vi "UpdateCurveSetup.vi"(8 "ErrorIn(No Error)":errorcluster caption="entrée d'erreur (pas d'erreur)", 10 "CurveSetupsIn":T1[](array[typedef]), 11 "Interface.lvclass":refnum<class "Interface.lvclass">) -> (0 "sortie d'erreur":errorcluster, 3 "Interface.lvclass Out":refnum<class "Interface.lvclass">)   [LabVIEW 2019, in "Interface.lvclass"]
uses:
  Interface.lvclass
  CurveSetup.ctl
  Interface.lvclass/Interface.ctl
panel:
  # "Chemin de sauvegarde"
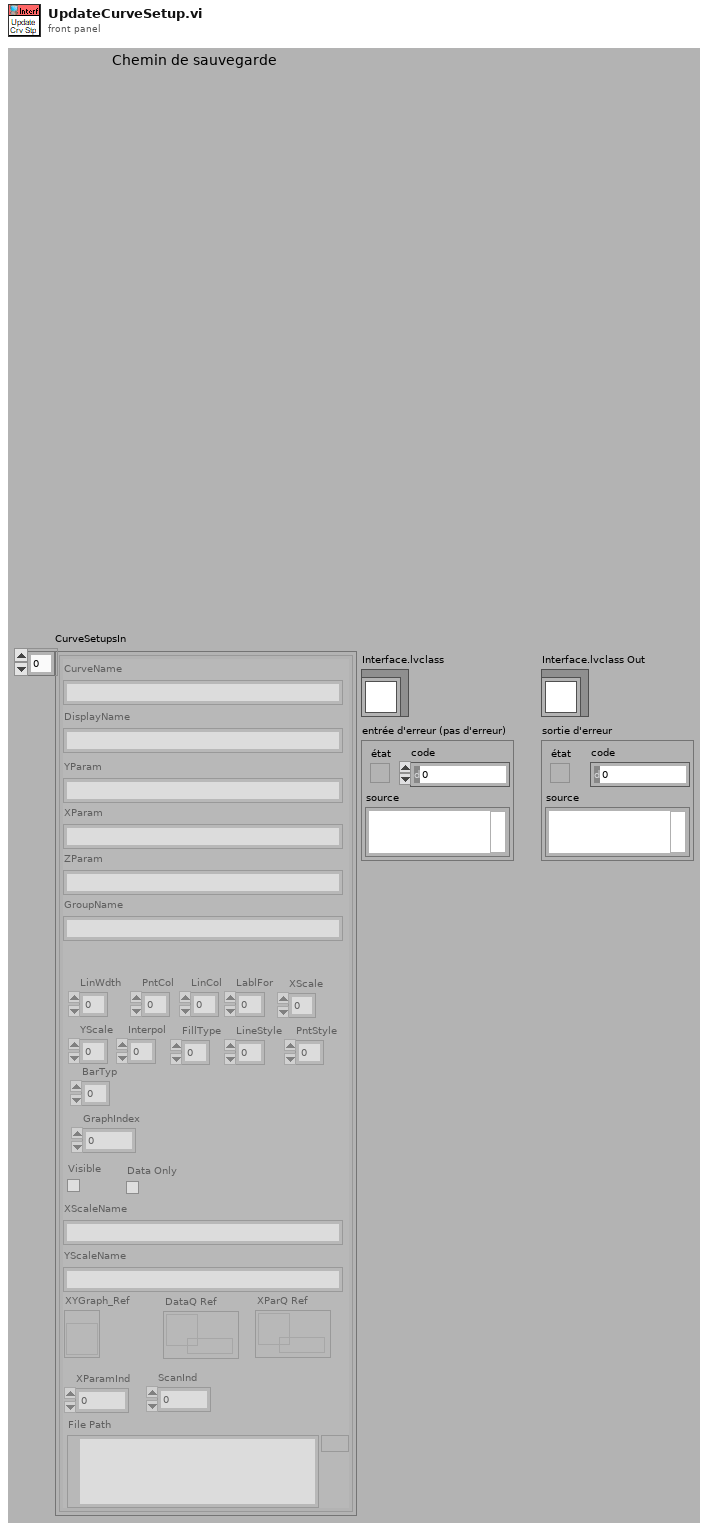
[diagram p1: front panel]
types:
  T1 = typedef "Interface.lvclass/CurveSetup.ctl" = cluster{"CurveName":string, "YParam":string, "XParam":string, "ZParam ":string, "GroupName":string, "LinWdth":u8, "PntCol":u32, "LinCol":u32, "LablFor":u8, "XScale":u32, "YScale":u32, "Interpol":u8, "DisplayName":string, "FillType":i16, "LineStyle":u8, "PntStyle":u8, "BarTyp":u8, "GraphIndex":i32, "Visible":bool, "XScaleName":string, "YScaleName":string, "XYGraph_Ref":refnum<vi>, "Data Only":bool, "DataQ Ref":refnum<queue>, "XParQ Ref":refnum<queue>, "XParamInd":i32, "ScanInd":i32, "File Path":path}
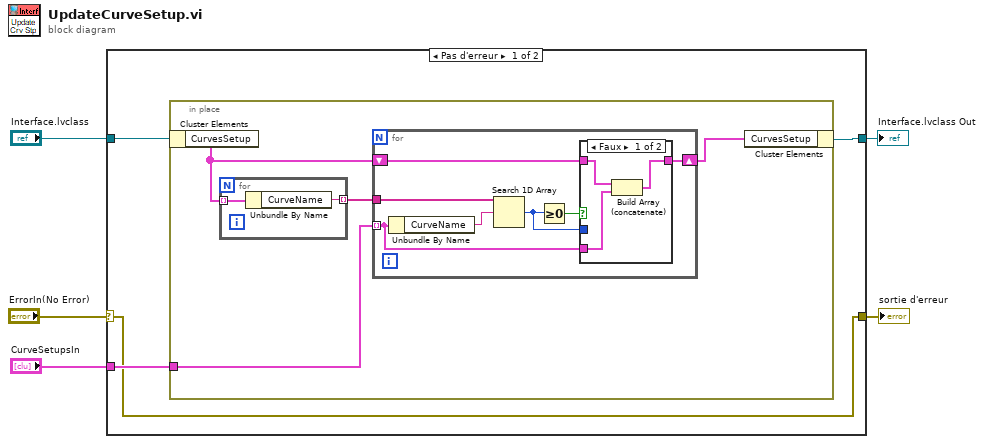
[diagram p0: block diagram]
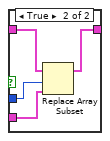
[diagram p2: hidden frame]
diagram:
  n1 = case shown="Pas d'erreur" "ErrorIn(No Error)" {
    selector: "ErrorIn(No Error)" -> [w6 w31]
    tunnel: [w6 w31] -> w4
    tunnel: "Interface.lvclass" -> [w9 w30]
    tunnel: [w7 w30] -> w2
    tunnel: "CurveSetupsIn" -> [w8 _]
    frame No Error {
      n2 = in-place {
        in-place-border: w8 -> [w11]
        n3 = in-place-cluster #1(w9) -> ("CurvesSetup"=w13:T1[])
        n4 = for {
          tunnel: w13 -> [w15] mode=indexing
          tunnel: [w14] -> w12 mode=indexing
          n5 = Unbundle By Name(w15) -> ("CurveName"=w14:string)
        }
        n6 = for {
          tunnel: w11 -> [w18] mode=indexing
          shift-right: [w19] -> w10
          shift-left: w13 -> [w20]
          tunnel: w12 -> [w22]
          n7 = Unbundle By Name(w18) -> ("CurveName"=w21:string)
          n8 = Search 1D Array(1D array=w22, element=w21) -> (index of element=w16:i32)  [unwired: 1 in]
          n9 = Greater Or Equal To 0?(x=w16) -> (x >= 0?=w17:bool)
          n10 = case shown="Faux" w17 {
            tunnel: w20 -> [w24 w29]
            tunnel: [w23 w28] -> w19
            tunnel: w18 -> [w25 w27]
            tunnel: w16 -> [_ w26]
            frame False {
              n11 = Build Array (concatenate)(w24, w25) -> (w23:T1[])
            }
            frame True {
              n12 = Replace Array Subset(array=w29, new element=w27, index=w26) -> (w28:T1[])
            }
          }
        }
        n13 = in-place-cluster #1("CurvesSetup"=w10) -> (w7:refnum<class "Interface.lvclass">)
      }
    }
    frame Error {
    }
  }
  "sortie d'erreur" <- w4
  "Interface.lvclass Out" <- w2
